vi "Pixy_COM-PC.vi"() -> ()   [LabVIEW 2015]
uses:
  <vilib>/Analysis/baseanly.llb/Mean (DBL).vi
  <vilib>/Instr/_visa.llb/VISA Configure Serial Port (Instr).vi
  <vilib>/Analysis/NI_AALBase.lvlib
panel:
  out "Data display":string
  in  "Display buffer size":u16=100 min=1
  in  "Write Command?":bool
  in  "Command":string(combo)
  out "Area":dbl(graph)
  out "Height":i32
  out "Width":i32
  out "Y":i32
  out "X":i32
  out "Read error out":errorcluster
  out "Initialization error out":errorcluster
  in  "stop":bool
  in  "VISA resource name":refnum<visa-resource-name>="COM3"
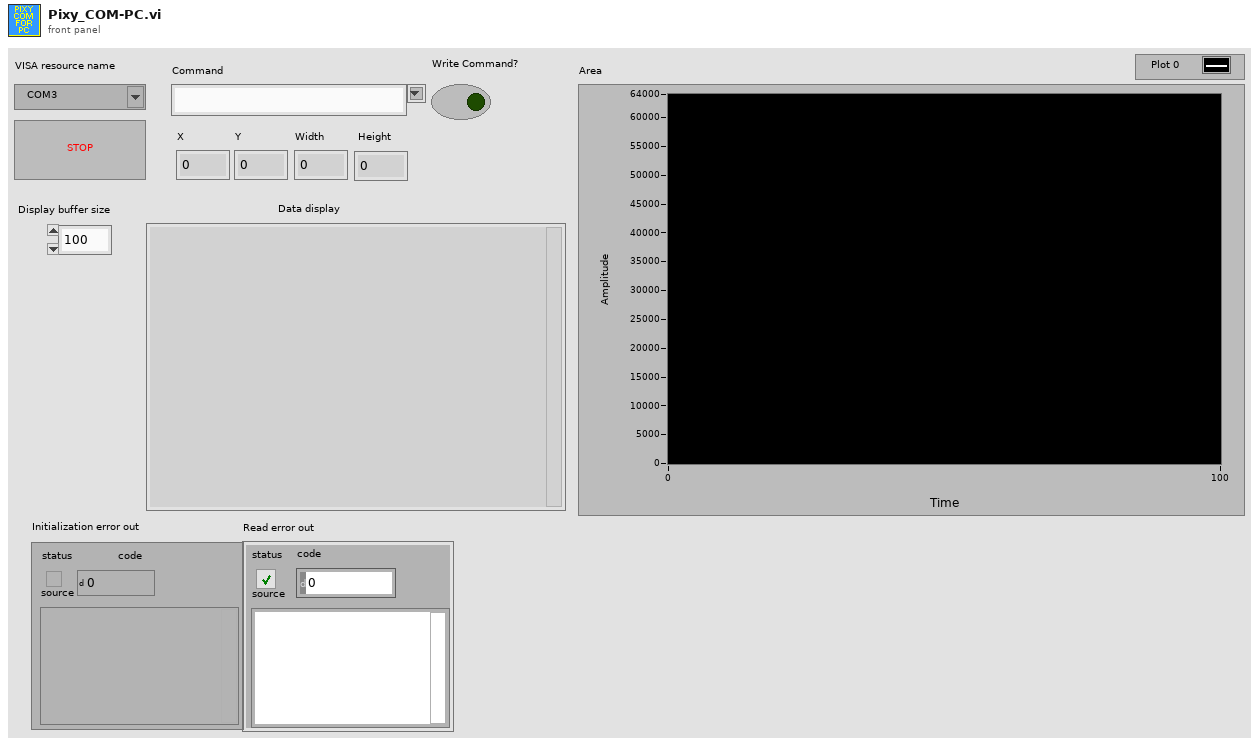
[diagram p1: front panel]
types:
  T1 = cluster{"buffer":string, "X":i32, "Y":i32, "Width":i32, "Height":i32, "Area":dbl}
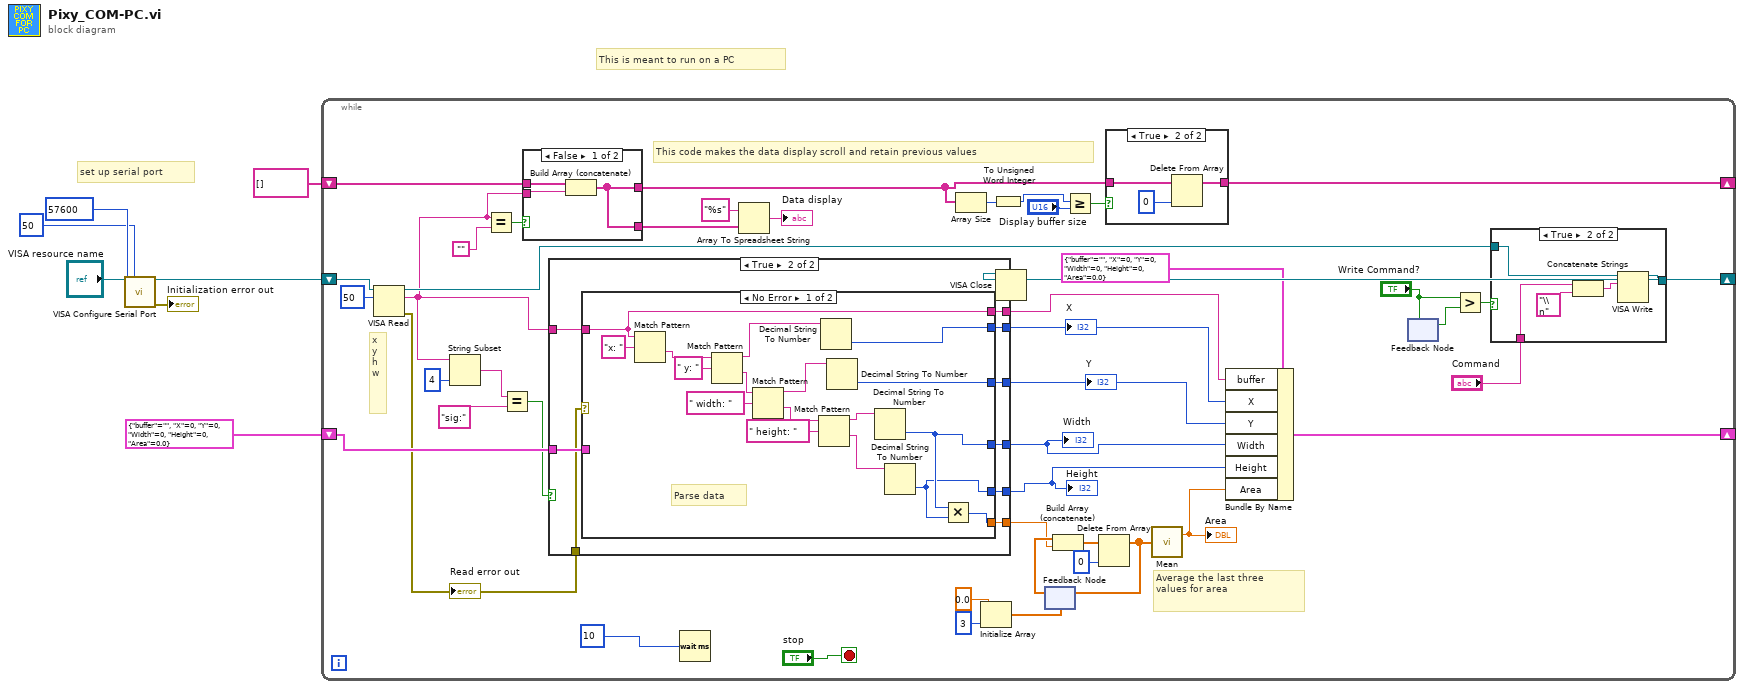
[diagram p0: block diagram]
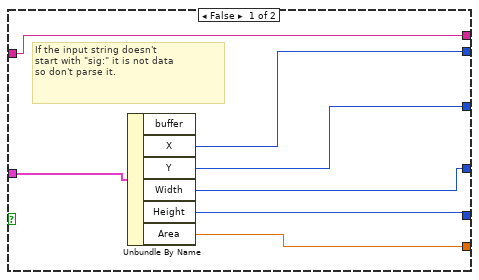
[diagram p4: hidden frame]
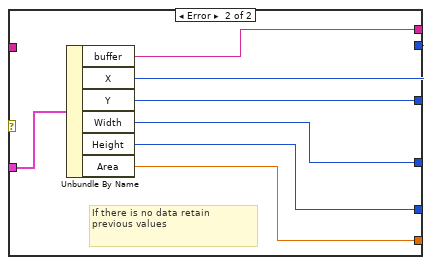
[diagram p5: hidden frame]
diagram:
  # "set up serial port"
  # "This is meant to run on a PC"
  n1 = call-poly "VISA Configure Serial Port"("VISA resource name"="VISA resource name", "timeout (10sec)"=u32 50, "baud rate (9600)"=u32 57600) -> ("VISA resource name out"=w2:refnum<visa-resource-name>, "error out"=→"Initialization error out":errorcluster)  [unwired: 11 in]
  n2 = while {
    shift-right: [w39] -> w8
    shift-left: w2 -> [w50]
    shift-right: [w49] -> _
    shift-left: T1 {"buffer"="", "X"=0, "Y"=0, "Width"=0, "Height"=0, "Area"=0.0} -> [w33]
    shift-right: [w16] -> _
    shift-left: string[] [] -> [w22]
    stop <- "stop" stop-if-true
    # "Average the last three\nvalues for area"
    # "This code makes the data display scroll and retain previous values"
    # "x\ny\nh\nw"
    n3 = VISA Read(VISA resource name=w50, byte count=u32 50) -> (VISA resource name out=w40:refnum<visa-resource-name>, read buffer=w12:string, error out=w28:errorcluster)  [unwired: 1 in, 1 out]
    "Read error out" <- w28
    n4 = String Subset(string=w12, length (rest)=4 ("length (rest)")) -> (substring=w29:string)  [unwired: 1 in]
    n5 = Equal?(x=w12, y="") -> (x = y?=w13:bool)
    n6 = Equal?(x=w29, y="sig:") -> (x = y?=w31:bool)
    n7 = case shown="False" w13 {
      tunnel: w22 -> [w54 w57]
      tunnel: [w56 w57] -> w17
      tunnel: [w56 w57] -> w14
      tunnel: w12 -> [w55 _]
      frame False {
        n8 = Build Array (concatenate)(w54, w55) -> (w56:string[])
      }
      frame True {
      }
    }
    n9 = case shown="True" w31 {
      tunnel: [w62 w77] -> w38
      tunnel: [w67 w76] -> w37
      tunnel: [w66 w75] -> w36
      tunnel: [w65 w74] -> w35
      tunnel: [w64 w73] -> w9
      tunnel: [w63 w72] -> w34
      tunnel: w12 -> [w62 w71]
      tunnel: w33 -> [w68 w70]
      tunnel: w28 -> [_ w69]
      frame False {
        # "If the input string doesn't\nstart with \"sig:\" it is not data\nso don't parse it."
        n10 = Unbundle By Name(w68) -> ("X"=w67:i32, "Y"=w66:i32, "Width"=w65:i32, "Height"=w64:i32, "Area"=w63:dbl)  [unwired: 1 out]
      }
      frame True {
        n11 = case shown="No Error" w69 {
          tunnel: [w90 w96] -> w76
          tunnel: [w86 w97] -> w75
          tunnel: [w81 w98] -> w74
          tunnel: [w80 w99] -> w73
          tunnel: [w79 w100] -> w72
          tunnel: w70 -> [_ w101]
          tunnel: w71 -> [w78 _]
          tunnel: [w78 w95] -> w77
          frame No Error {
            # "Parse data"
            n12 = Match Pattern(string=w78, regular expression="x: ") -> (after substring=w93:string)  [unwired: 1 in, 3 out]
            n13 = Match Pattern(string=w93, regular expression=" y: ") -> (before substring=w91:string, after substring=w89:string)  [unwired: 1 in, 2 out]
            n14 = Match Pattern(string=w89, regular expression=" width: ") -> (before substring=w87:string, after substring=w85:string)  [unwired: 1 in, 2 out]
            n15 = Match Pattern(string=w85, regular expression=" height: ") -> (before substring=w83:string, after substring=w82:string)  [unwired: 1 in, 2 out]
            n16 = Decimal String To Number(string=w91) -> (number=w90:i32)  [unwired: 2 in, 1 out]
            n17 = Decimal String To Number(string=w87) -> (number=w86:i32)  [unwired: 2 in, 1 out]
            n18 = Decimal String To Number(string=w83) -> (number=w81:i32)  [unwired: 2 in, 1 out]
            n19 = Decimal String To Number(string=w82) -> (number=w80:i32)  [unwired: 2 in, 1 out]
            n20 = Multiply(x=w81, y=w80) -> (x*y=w79:i32)
          }
          frame Error {
            # "If there is no data retain \nprevious values"
            n21 = Unbundle By Name(w101) -> ("buffer"=w95:string, "X"=w96:i32, "Y"=w97:i32, "Width"=w98:i32, "Height"=w99:i32, "Area"=w100:dbl)
          }
        }
      }
    }
    "X" <- w37
    "Y" <- w36
    "Width" <- w35
    "Height" <- w9
    n22 = Wait (ms)(milliseconds to wait=u32 10) -> ()  [unwired: 1 out]
    n23 = Array To Spreadsheet String(array=w17, 3:"%s" ("format string")) -> (spreadsheet string=→"Data display":string)  [unwired: 1 in]
    n24 = Array Size(array=w14) -> (size(s)=w19:i32)
    n25 = Initialize Array(0.0 ("element"), 3 ("dimension size")) -> (w45:dbl[])
    n26 = To Unsigned Word Integer(number=w19) -> (unsigned 16bit integer=w18:u16)
    n27 = feedback #1(w45) -> (w41:dbl[])
    n28 = Build Array (concatenate)(w41, w34) -> (w44:dbl[])
    n29 = Greater Or Equal?(x=w18, y="Display buffer size") -> (x >= y?=w15:bool)
    n30 = Delete From Array(array=w44, index=0) -> (array with subset deleted=w43:dbl[])  [unwired: 1 in, 1 out]
    n31 = feedback-in #1(w43) -> ()
    n32 = case shown="True" w15 {
      tunnel: w14 -> [w58 w61]
      tunnel: [w58 w60] -> w16
      frame False {
      }
      frame True {
        n33 = Delete From Array(array=w61, index=0) -> (array with subset deleted=w60:string[])  [unwired: 1 in, 1 out]
      }
    }
    n34 = call-poly <vilib>:"Mean.vi"("X"=w43) -> ("mean"=w48:dbl)  [unwired: 1 out]
    "Area" <- w48
    n35 = Bundle By Name(cluster=T1 {"buffer"="", "X"=0, "Y"=0, "Width"=0, "Height"=0, "Area"=0.0}, "buffer"=w38, "X"=w37, "Y"=w36, "Width"=w35, "Height"=w9, "Area"=w48) -> (w49:T1)
    n36 = feedback-in #2("Write Command?") -> ()
    n37 = feedback #2() -> (w25:bool)  [unwired: 1 in]
    n38 = Greater?(x="Write Command?", y=w25) -> (0:w26:bool)
    n39 = case shown="True" w26 {
      tunnel: w40 -> [w102 w107]
      tunnel: [w102 w106] -> w39
      tunnel: "Command" -> [_ w104]
      frame False {
      }
      frame True {
        n40 = Concatenate Strings(w104, "\\n") -> (w105:string)
        n41 = VISA Write(VISA resource name=w107, write buffer=w105) -> (VISA resource name out=w106:refnum<visa-resource-name>)  [unwired: 1 in, 2 out]
      }
    }
  }
  n42 = VISA Close(VISA resource name=w8) -> ()  [unwired: 1 in, 1 out]
